vi "LIA Example FPGA_Original.vi"() -> ()   [LabVIEW 2017]
uses:
  <vilib>/eio/EIONode/EIONode.xnode
  <vilib>/rvi/eio/common/nirviEmuTemplateMethod_errors.vi
  <vilib>/Platform/TimedLoop/XDataNode/wakeup.ctl
  <vilib>/Platform/TimedLoop/XDataNode/XDNodeRunTimeDep.lvlib
  <vilib>/Platform/TimedLoop/XDataNode/nitl_modes.ctl
  <vilib>/Platform/TimedLoop/XDataNode/timing_clust.ctl
  <vilib>/Platform/TimedLoop/XDataNode/XDataNode.xnode
  <instrlib>/_niInstr/Basic Elements/v1/FPGA/niInstr Basic Elements v1 FPGA.lvlib
  <instrlib>/_niInstr/DSP/v1/Shared/Public/IQ Data.ctl
  <instrlib>/_niInstr/DSP/v1/Shared/niInstr DSP v1 Shared.lvlib
  <instrlib>/_niInstr/DSP/v1/FPGA/Public/Sub VIs/Frequency Shift/Frequency Shift - 1 spc.vi
  <instrlib>/_niInstr/DSP/v1/FPGA/niInstr DSP v1 FPGA.lvlib
  <instrlib>/_niInstr/DSP/v1/Xnodes/Public/Frequency Shift/niInstr DSP v1 Frequency Shift FPGA.xnode
  Program Files (x86)/National Instruments/LabVIEW 2017/examples/Lock-In Amplifier/_NI PLL IP/FPGA/NI PLL IP FPGA.lvlib
  <vilib>/rvi/FXPMathLib/FxpMul/XNode/nifxpmath_Multiplier.xnode
  <vilib>/rvi/FXPMathLib/FxpAdd/XNode/nifxpmath_Add.xnode
  <instrlib>/_niInstr/DSP/v1/FPGA/Public/Sub VIs/Frequency Shift/Frequency Shift - 2 spc.vi
  Program Files (x86)/National Instruments/LabVIEW 2017/examples/Lock-In Amplifier/lib/fpga/Lock-In Amplifier Example FPGA.lvlib
  <instrlib>/_niInstr/Streaming/v1/Common/Stream State.ctl
  <instrlib>/_niInstr/Streaming/v1/Common/niInstr Streaming v1 Common.lvlib
  <userlib>/_NI Noise Generation IP/FPGA/NI Noise Generation IP FPGA v2.lvlib
  <vilib>/rvi/FXPMathLib/sim/FxpSim.dll
  <userlib>/_NI Noise Generation IP/FPGA/Public/Low Level/AWGN FXP23x2.vi
panel:
  in  "lock-in.enable 3":bool
  in  "lock-in.enable 2":bool
  in  "lock-in.enable 1":bool
  in  "lock-in.carrier 3":fxp<+/-,48,0>
  in  "lock-in.carrier 2":fxp<+/-,48,0>
  in  "lock-in.enable 0":bool
  in  "lock-in.channel select 3":i32
  in  "lock-in.carrier select 3":i32
  in  "lock-in.cic config valid 3":bool
  in  "lock-in.cic config 3":cluster{"factor":fxp<+,16,16>, "shift":i16}
  in  "lock-in.reset 3":bool
  out "stream.state 3":T1 caption="stream.state 0"
  out "stream.samples transferred 3":u64 caption="stream.samples transferred 0"
  out "stream.metadata 3":u64 caption="stream.metadata 0"
  in  "stream.num samples 3":u64 caption="stream.num samples 0"
  in  "stream.request state 3":T1 caption="stream.request state 0"
  in  "lock-in.channel select 2":i32
  in  "lock-in.carrier select 2":i32
  in  "lock-in.cic config valid 2":bool
  in  "lock-in.cic config 2":cluster{"factor":fxp<+,16,16>, "shift":i16}
  in  "lock-in.reset 2":bool
  out "stream.state 2":T1 caption="stream.state 0"
  out "stream.samples transferred 2":u64 caption="stream.samples transferred 0"
  out "stream.metadata 2":u64 caption="stream.metadata 0"
  in  "stream.num samples 2":u64 caption="stream.num samples 0"
  in  "stream.request state 2":T1 caption="stream.request state 0"
  out "pll.vco output 0":fxp<+/-,48,0>
  out "pll.vco output 1":fxp<+/-,48,0>
  out "stream.metadata 4":u64 caption="stream.metadata 0"
  out "stream.samples transferred 4":u64 caption="stream.samples transferred 0"
  out "stream.state 4":T1 caption="stream.state 0"
  in  "stream.request state 4":T1 caption="stream.request state 0"
  in  "stream.num samples 4":u64 caption="stream.num samples 0"
  in  "preview.channel select":i32
  in  "ao.reset 3":bool
  in  "ao.carrier 2":fxp<+/-,48,0>=0.010000000000001563
  in  "ao.level 2":fxp<+/-,18,1>
  in  "ao.reset 2":bool
  in  "ao.carrier 1":fxp<+/-,48,0>=0.010000000000001563
  in  "ao.level 1":fxp<+/-,18,1>
  in  "ao.reset 1":bool
  in  "ao.reset 0":bool
  in  "ao.carrier 0":fxp<+/-,48,0>=0.010000000000001563
  in  "ao.level 0":fxp<+/-,18,1>
  in  "lock-in.channel select 1":i32
  in  "lock-in.channel select 0":i32
  in  "stream.request state 1":T1 caption="stream.request state 0"
  in  "stream.num samples 1":u64 caption="stream.num samples 0"
  out "stream.metadata 1":u64 caption="stream.metadata 0"
  out "stream.samples transferred 1":u64 caption="stream.samples transferred 0"
  out "stream.state 1":T1 caption="stream.state 0"
  in  "lock-in.reset 1":bool
  in  "lock-in.cic config 1":cluster{"factor":fxp<+,16,16>, "shift":i16}
  in  "lock-in.cic config valid 1":bool
  in  "lock-in.carrier select 1":i32
  in  "lock-in.carrier select 0":i32
  in  "lock-in.cic config valid 0":bool
  in  "lock-in.cic config 0":cluster{"factor":fxp<+,16,16>, "shift":i16}
  in  "lock-in.reset 0":bool
  in  "lock-in.carrier 1":fxp<+/-,48,0>
  in  "lock-in.carrier 0":fxp<+/-,48,0>
  in  "ao.level 3":fxp<+/-,18,1>
  in  "pll.channel 1":i32
  in  "pll.reset 1":bool
  in  "pll.enable 1":bool
  in  "pll.config 1":T2={"quiescent frequency"=0.10000000000000142, "compensation"=0.0, "psd gain"=-18, "loop filter"={"order"=4, "cutoff"=6}}
  in  "pll.channel 0":i32
  in  "ao.noise gain 3":fxp<+,18,1>=0.01000213623046875
  in  "ao.carrier 3":fxp<+/-,48,0>=0.010000000000001563
  in  "ao.noise seeds 3":fxp<+,23,23>[](array[numeric])=[1.0, 12323.0]
  in  "pll.reset 0":bool
  in  "pll.enable 0":bool
  in  "stream.request state 0":T1
  in  "stream.num samples 0":u64
  out "stream.metadata 0":u64
  out "stream.samples transferred 0":u64
  out "stream.state 0":T1
  in  "pll.config 0":T2={"quiescent frequency"=0.10000000000000142, "compensation"=0.0, "psd gain"=-18, "loop filter"={"order"=4, "cutoff"=6}}
  out "IO Module\\InitDone":bool
  out "IO Module\\User Error":u32
  in  "IO Module\\User Command":u32
  in  "IO Module\\User Command Valid":bool
  out "IO Module\\User Command Ready":bool
  in  "IO Module\\User Command Arg 0":u32
  in  "IO Module\\User Command Arg 1":u32
  out "IO Module\\User Command Error":u16
  out "IO Module\\User Command Return":u32
  out "IO Module\\User Command Return Valid":bool
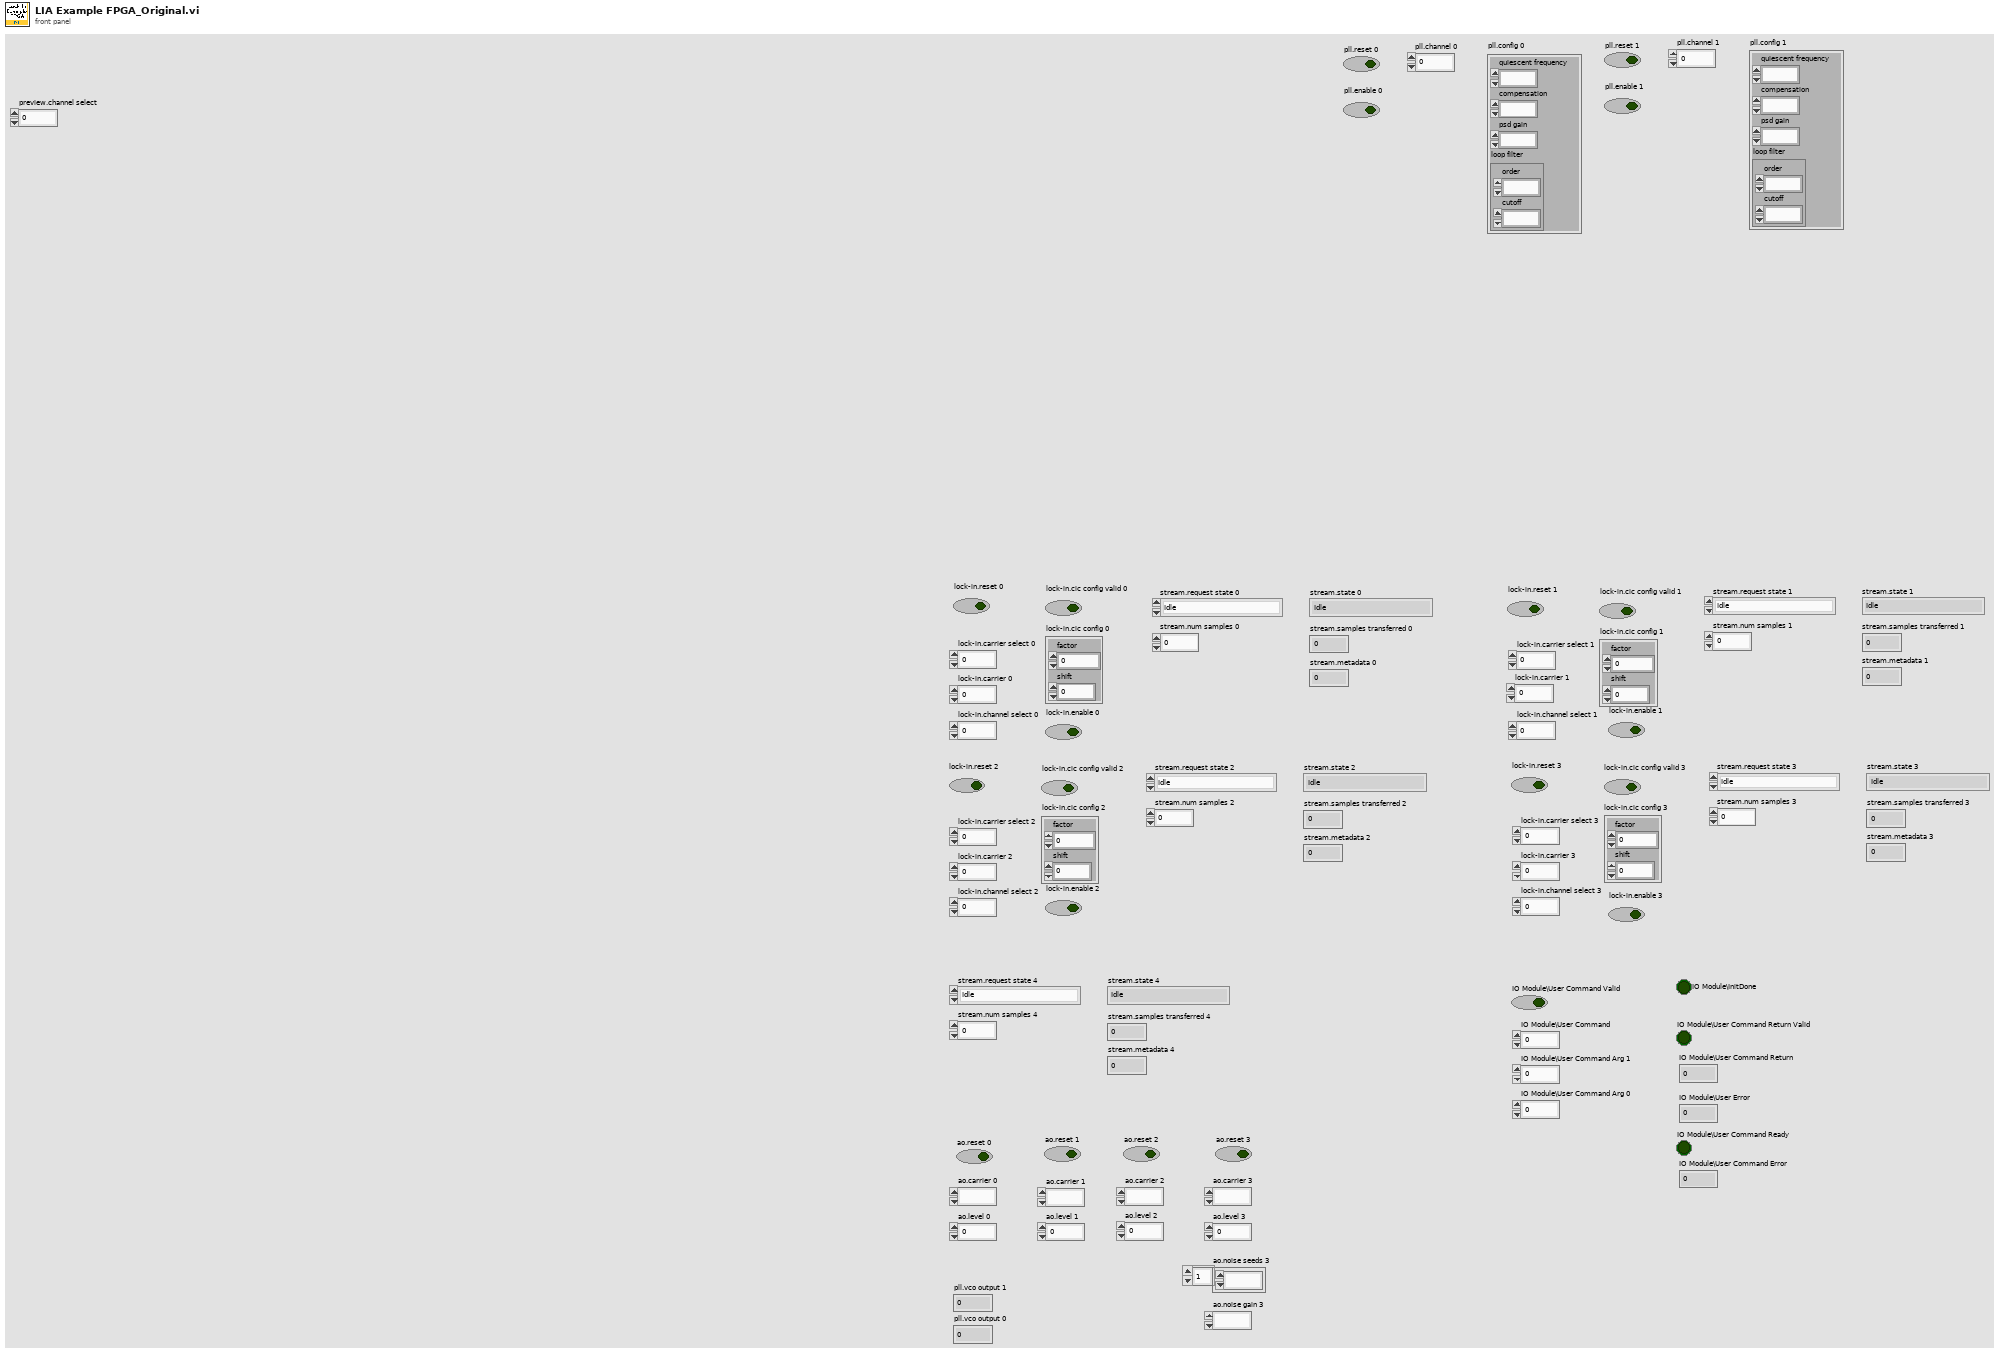
[diagram p1: front panel]
types:
  T1 = typedef "niInstr Streaming v1 Common.lvlib/Stream State.ctl" = enum8{"Idle", "Finite Transfer", "Continuous", "Done", "Error", "Not Ready", "Cancel"}
  T2 = cluster{"quiescent frequency":fxp<+/-,48,0>, "compensation":fxp<+/-,18,3>, "psd gain":i16, "loop filter":cluster{"order":i32, "cutoff":i8}}
  T3 = typedef "XDNodeRunTimeDep.lvlib/timing_clust.ctl" = cluster{"Expected End [f-1]":u64, "Actual End [f-1]":u64, "Finished Late? [f-1]":bool, "Expected End [i-1]":u64, "Actual End [i-1]":u64, "Finished Late? [i-1]":bool, "Expected Start [i]":u64, "Actual Start [i]":u64, "Expected Start [f]":u64, "Actual Start [f]":u64, "Source Name":string, "Structure Name":string, "Period":i64, "Deadline":i64, "Offset":i64, "Start":i64, "Priority":i32, "Timeout":i32, "Mode":T4, "Wakeup Reason":T5, "Error":errorcluster, "Source Type":string, "Secondary Source Type":string, "Global End Time":u64, "Global Start Time":u64, "Frame Duration":u64, "Iteration Duration":u64, "Assigned CPU":i32, "I/O Scan Engine Mode":u32}
  T4 = typedef "XDNodeRunTimeDep.lvlib/nitl_modes.ctl" = enum32{"No Change", "Process missed periods, maintain original phase", "Discard missed periods, maintain original phase", "Process missed periods, ignore original phase", "Discard missed periods, ignore original phase"}
  T5 = typedef "XDNodeRunTimeDep.lvlib/wakeup.ctl" = enum32{"Normal", "Aborted", "Asynchronous wakeup", "Timing source error", "Timed loop error", "Timeout"}
  T6 = cluster{"stream.num samples 0":u64, "stream.request state 0":T1, "stream.index 0":i16}
  T7 = typedef "niInstr DSP v1 Shared.lvlib/IQ Data.ctl" = cluster{"I":fxp<+/-,18,1>, "Q":fxp<+/-,18,1>, "overflow":bool}
  T8 = cluster{"stream.metadata 0":u64, "stream.samples transferred 0":u64, "stream.state 0":T1}
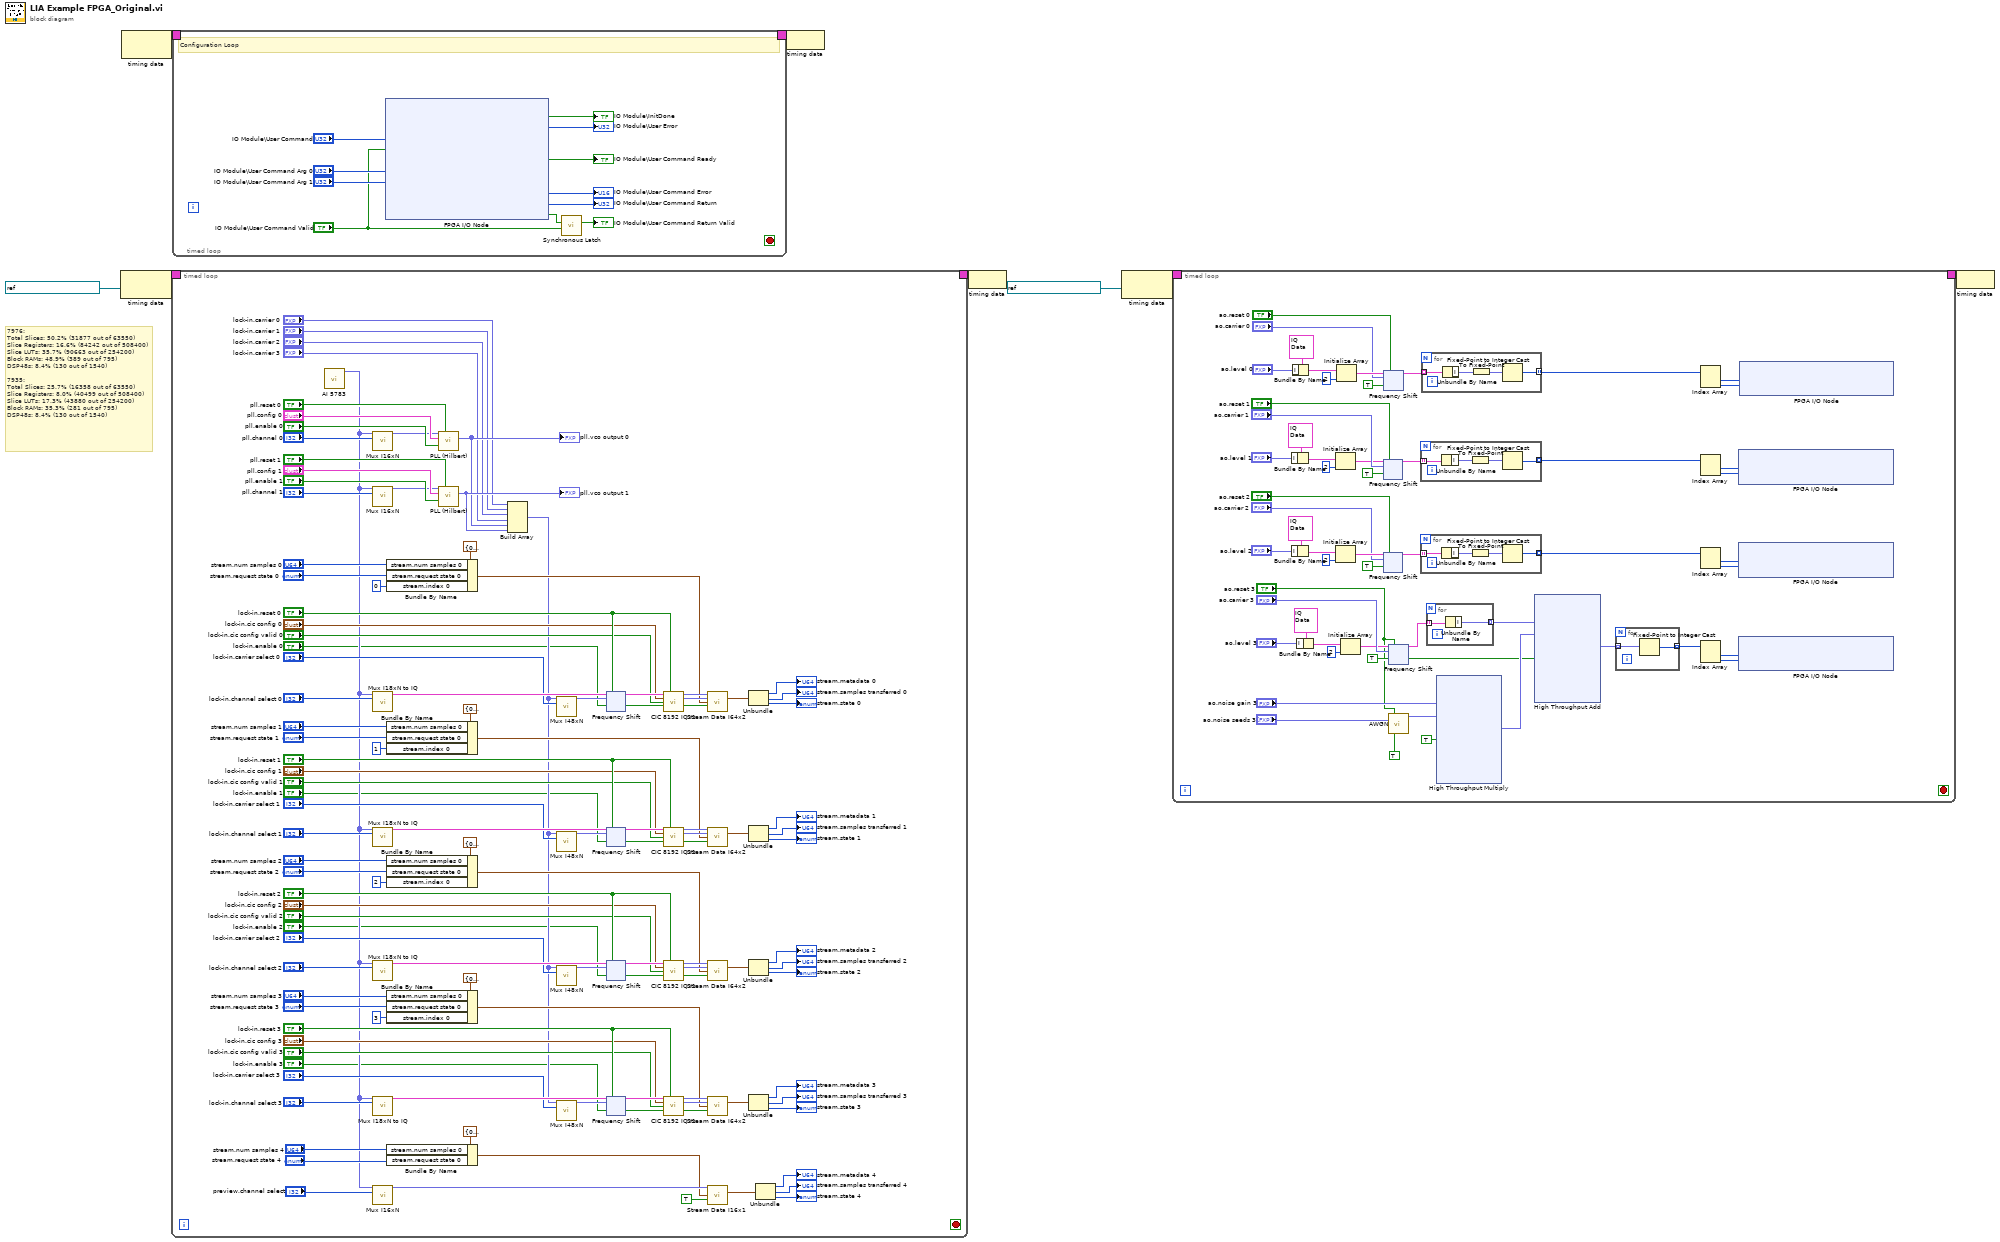
[diagram p0: block diagram]
diagram:
  # "7976:\nTotal Slices: 50.2% (31877 out of 63550)\nSlice Registers: 16.6% (84242 out of 508400)\nSlice LUTs: 35.7% (90663 out of 254200)\nBlock RAMs: 48.9% (389 out of 795)\nDSP48s: 8.4% (130 out of 1540)\n\n7935:\nTotal Slices: 25.7% (16358 out of 63550)\nSlice Registers: 8.0% (40499 out of 508400)\nSlice LUTs: 17.3% (43880 out of 254200)\nBlock RAMs: 35.3% (281 out of 795)\nDSP48s: 8.4% (130 out of 1540)"
  n1 = node-c288(refnum<k21> "IO Module\\Data Clock" ("Source Name")) -> (w8:T3)
  n2 = node-c288() -> (w2:T3)  [unwired: 1 in]
  n3 = timed-loop {
    timing: w8 -> [_]
    timing-out: [_] -> w7
    stop <- _ stop-if-true
    n4 = call "AI 5783.vi"() -> ("i18x1"=w17:fxp<+/-,18,1>[])  [unwired: 14 in, 1 out]
    n5 = call "Mux I16xN.vi"("i16xn in"=w17, "index"="pll.channel 0") -> ("i16 out"=w122:fxp<+/-,18,1>)  [unwired: 12 in, 1 out]
    n6 = call "Mux I16xN.vi"("i16xn in"=w17, "index"="pll.channel 1") -> ("i16 out"=w116:fxp<+/-,18,1>)  [unwired: 12 in, 1 out]
    n7 = call "Mux I18xN to IQ.vi"("i16xn in"=w17, "index"="lock-in.channel select 0") -> ("output"=w115:T7)  [unwired: 12 in, 1 out]
    n8 = call "Mux I18xN to IQ.vi"("i16xn in"=w17, "index"="lock-in.channel select 1") -> ("output"=w94:T7)  [unwired: 12 in, 1 out]
    n9 = call "Mux I18xN to IQ.vi"("i16xn in"=w17, "index"="lock-in.channel select 2") -> ("output"=w60:T7)  [unwired: 12 in, 1 out]
    n10 = call "Mux I18xN to IQ.vi"("i16xn in"=w17, "index"="lock-in.channel select 3") -> ("output"=w39:T7)  [unwired: 12 in, 1 out]
    n11 = call "Mux I16xN.vi"("i16xn in"=w17, "index"="preview.channel select") -> ("i16 out"=w68:fxp<+/-,18,1>)  [unwired: 12 in, 1 out]
    n12 = Bundle By Name(cluster=T6 {"stream.num samples 0"=0, "stream.request state 0"=enum."Idle", "stream.index 0"=0} ("config"), "stream.num samples 0"="stream.num samples 0", "stream.request state 0"="stream.request state 0", "stream.index 0"=i16 0) -> (w97:T6)
    n13 = Bundle By Name(cluster=T6 {"stream.num samples 0"=0, "stream.request state 0"=enum."Idle", "stream.index 0"=0} ("config"), "stream.num samples 0"="stream.num samples 1", "stream.request state 0"="stream.request state 1", "stream.index 0"=i16 1) -> (w76:T6)
    n14 = Bundle By Name(cluster=T6 {"stream.num samples 0"=0, "stream.request state 0"=enum."Idle", "stream.index 0"=0} ("config"), "stream.num samples 0"="stream.num samples 2", "stream.request state 0"="stream.request state 2", "stream.index 0"=i16 2) -> (w42:T6)
    n15 = Bundle By Name(cluster=T6 {"stream.num samples 0"=0, "stream.request state 0"=enum."Idle", "stream.index 0"=0} ("config"), "stream.num samples 0"="stream.num samples 3", "stream.request state 0"="stream.request state 3", "stream.index 0"=i16 3) -> (w21:T6)
    n16 = Bundle By Name(cluster=T6 {"stream.num samples 0"=0, "stream.request state 0"=enum."Idle", "stream.index 0"=0} ("config"), "stream.num samples 0"="stream.num samples 4", "stream.request state 0"="stream.request state 4") -> (w64:T6)
    n17 = call "PLL (Hilbert).vi"("input"=w122, "reset"="pll.reset 0", "config"="pll.config 0", "enable"="pll.enable 0") -> ("output"=w61:fxp<+/-,48,0>)  [unwired: 11 in]
    "pll.vco output 0" <- w61
    n18 = call "PLL (Hilbert).vi"("input"=w116, "reset"="pll.reset 1", "config"="pll.config 1", "enable"="pll.enable 1") -> ("output"=w62:fxp<+/-,48,0>)  [unwired: 11 in]
    "pll.vco output 1" <- w62
    n19 = Build Array("lock-in.carrier 0", "lock-in.carrier 1", "lock-in.carrier 2", "lock-in.carrier 3", w61, w62) -> (w18:fxp<+/-,48,0>[])
    n20 = call "Mux I48xN.vi"("i48xn in"=w18, "index"="lock-in.carrier select 0") -> ("i48 out"=w114:fxp<+/-,48,0>)  [unwired: 13 in]
    n21 = call "Mux I48xN.vi"("i48xn in"=w18, "index"="lock-in.carrier select 1") -> ("i48 out"=w93:fxp<+/-,48,0>)  [unwired: 13 in]
    n22 = call "Mux I48xN.vi"("i48xn in"=w18, "index"="lock-in.carrier select 2") -> ("i48 out"=w59:fxp<+/-,48,0>)  [unwired: 13 in]
    n23 = call "Mux I48xN.vi"("i48xn in"=w18, "index"="lock-in.carrier select 3") -> ("i48 out"=w38:fxp<+/-,48,0>)  [unwired: 13 in]
    n24 = xnode "Frequency Shift"("data in"=w115, "reset"="lock-in.reset 0", "frequency shift"=w114, "input valid"="lock-in.enable 0") -> ("data out"=w113:T7, "output valid"=w112:bool)  [unwired: 2 in, 1 out]
    n25 = xnode "Frequency Shift"("data in"=w94, "reset"="lock-in.reset 1", "frequency shift"=w93, "input valid"="lock-in.enable 1") -> ("data out"=w92:T7, "output valid"=w91:bool)  [unwired: 2 in, 1 out]
    n26 = xnode "Frequency Shift"("data in"=w60, "reset"="lock-in.reset 2", "frequency shift"=w59, "input valid"="lock-in.enable 2") -> ("data out"=w58:T7, "output valid"=w57:bool)  [unwired: 2 in, 1 out]
    n27 = xnode "Frequency Shift"("data in"=w39, "reset"="lock-in.reset 3", "frequency shift"=w38, "input valid"="lock-in.enable 3") -> ("data out"=w37:T7, "output valid"=w36:bool)  [unwired: 2 in, 1 out]
    n28 = call "CIC 8192 IQx1.vi"("data"=w113, "reset"="lock-in.reset 0", "config"="lock-in.cic config 0", "config valid"="lock-in.cic config valid 0", "input valid"=w112) -> ("i out"=w108:fxp<+/-,64,1>, "q out"=w107:fxp<+/-,64,1>, "output valid"=w106:bool)  [unwired: 8 in]
    n29 = call "CIC 8192 IQx1.vi"("data"=w92, "reset"="lock-in.reset 1", "config"="lock-in.cic config 1", "config valid"="lock-in.cic config valid 1", "input valid"=w91) -> ("i out"=w87:fxp<+/-,64,1>, "q out"=w86:fxp<+/-,64,1>, "output valid"=w85:bool)  [unwired: 8 in]
    n30 = call "CIC 8192 IQx1.vi"("data"=w58, "reset"="lock-in.reset 2", "config"="lock-in.cic config 2", "config valid"="lock-in.cic config valid 2", "input valid"=w57) -> ("i out"=w53:fxp<+/-,64,1>, "q out"=w52:fxp<+/-,64,1>, "output valid"=w51:bool)  [unwired: 8 in]
    n31 = call "CIC 8192 IQx1.vi"("data"=w37, "reset"="lock-in.reset 3", "config"="lock-in.cic config 3", "config valid"="lock-in.cic config valid 3", "input valid"=w36) -> ("i out"=w32:fxp<+/-,64,1>, "q out"=w31:fxp<+/-,64,1>, "output valid"=w30:bool)  [unwired: 8 in]
    n32 = call "Stream Data I64x2.vi"("i in"=w108, "q in"=w107, "config"=w97, "input valid"=w106) -> ("status"=w105:T8)  [unwired: 11 in]
    n33 = call "Stream Data I64x2.vi"("i in"=w87, "q in"=w86, "config"=w76, "input valid"=w85) -> ("status"=w84:T8)  [unwired: 11 in]
    n34 = call "Stream Data I64x2.vi"("i in"=w53, "q in"=w52, "config"=w42, "input valid"=w51) -> ("status"=w50:T8)  [unwired: 11 in]
    n35 = call "Stream Data I64x2.vi"("i in"=w32, "q in"=w31, "config"=w21, "input valid"=w30) -> ("status"=w29:T8)  [unwired: 11 in]
    n36 = call "Stream Data I16x1.vi"("i in"=w68, "config"=w64, "input valid"=TRUE) -> ("status"=w70:T8)  [unwired: 12 in]
    n37 = Unbundle(w105) -> ("stream.metadata 0"=→"stream.metadata 0":u64, "stream.samples transferred 0"=→"stream.samples transferred 0":u64, "stream.state 0"=→"stream.state 0":T1)
    n38 = Unbundle(w84) -> ("stream.metadata 0"=→"stream.metadata 1":u64, "stream.samples transferred 0"=→"stream.samples transferred 1":u64, "stream.state 0"=→"stream.state 1":T1)
    n39 = Unbundle(w50) -> ("stream.metadata 0"=→"stream.metadata 2":u64, "stream.samples transferred 0"=→"stream.samples transferred 2":u64, "stream.state 0"=→"stream.state 2":T1)
    n40 = Unbundle(w29) -> ("stream.metadata 0"=→"stream.metadata 3":u64, "stream.samples transferred 0"=→"stream.samples transferred 3":u64, "stream.state 0"=→"stream.state 3":T1)
    n41 = Unbundle(w70) -> ("stream.metadata 0"=→"stream.metadata 4":u64, "stream.samples transferred 0"=→"stream.samples transferred 4":u64, "stream.state 0"=→"stream.state 4":T1)
  }
  n42 = timed-loop {
    timing: w2 -> [_]
    timing-out: [_] -> w1
    stop <- _ stop-if-true
    # "Configuration Loop"
    n43 = xnode "FPGA I/O Node"("IO Module\\User Command"="IO Module\\User Command", "IO Module\\User Command Valid"="IO Module\\User Command Valid", "IO Module\\User Command Arg 0"="IO Module\\User Command Arg 0", "IO Module\\User Command Arg 1"="IO Module\\User Command Arg 1") -> ("IO Module\\InitDone"=→"IO Module\\InitDone":bool, "IO Module\\Clip Error Code"=→"IO Module\\User Error":u32, "IO Module\\User Command Ready"=→"IO Module\\User Command Ready":bool, "IO Module\\User Command Error"=→"IO Module\\User Command Error":u16, "IO Module\\User Command Return"=→"IO Module\\User Command Return":u32, "IO Module\\User Command Return Valid"=w165:bool)  [unwired: 10 in, 10 out]
    n44 = call <instrlib>:"Synchronous Latch.vi"("clear"="IO Module\\User Command Valid", "set"=w165) -> ("out"=→"IO Module\\User Command Return Valid":bool)  [unwired: 9 in]
  }
  n45 = node-c288(w1) -> ()
  n46 = node-c288(w7) -> ()
  n47 = node-c288(refnum<k21> "IO Module\\Data Clock" ("Source Name")) -> (w5:T3)
  n48 = timed-loop {
    timing: w5 -> [_]
    timing-out: [_] -> w4
    stop <- _ stop-if-true
    n49 = Bundle By Name(cluster=T7 {"I"=0.0, "Q"=0.0, "overflow"=FALSE} ("output"), "I"="ao.level 1") -> (w198:T7)
    n50 = Bundle By Name(cluster=T7 {"I"=0.0, "Q"=0.0, "overflow"=FALSE} ("output"), "I"="ao.level 2") -> (w188:T7)
    n51 = Bundle By Name(cluster=T7 {"I"=0.0, "Q"=0.0, "overflow"=FALSE} ("output"), "I"="ao.level 0") -> (w213:T7)
    n52 = Bundle By Name(cluster=T7 {"I"=0.0, "Q"=0.0, "overflow"=FALSE} ("output"), "I"="ao.level 3") -> (w222:T7)
    n53 = Initialize Array(w198, 2 ("dimension size")) -> (w194:T7[])
    n54 = Initialize Array(w188, 2 ("dimension size")) -> (w192:T7[])
    n55 = Initialize Array(w213, 2 ("dimension size")) -> (w217:T7[])
    n56 = Initialize Array(w222, 2 ("dimension size")) -> (w218:T7[])
    n57 = xnode "Frequency Shift"("data in"=w194, "reset"="ao.reset 1", "frequency shift"="ao.carrier 1", "input valid"=TRUE) -> ("data out"=w202:T7[])  [unwired: 2 in, 2 out]
    n58 = xnode "Frequency Shift"("data in"=w192, "reset"="ao.reset 2", "frequency shift"="ao.carrier 2", "input valid"=TRUE) -> ("data out"=w184:T7[])  [unwired: 2 in, 2 out]
    n59 = xnode "Frequency Shift"("data in"=w217, "reset"="ao.reset 0", "frequency shift"="ao.carrier 0", "input valid"=TRUE) -> ("data out"=w209:T7[])  [unwired: 2 in, 2 out]
    n60 = xnode "Frequency Shift"("data in"=w218, "reset"="ao.reset 3", "frequency shift"="ao.carrier 3", "input valid"=TRUE) -> ("data out"=w233:T7[], "output valid"=w230:bool)  [unwired: 2 in, 1 out]
    n61 = call-poly <userlib>:"AWGN.vi"("reset"="ao.reset 3", "seeds"="ao.noise seeds 3", "ready"=TRUE) -> ("output 0"=w225:fxp<+/-,23,4>[])  [unwired: 10 in, 2 out]
    n62 = for {
      tunnel: w202 -> [w249] mode=indexing
      tunnel: [w250] -> w203 mode=indexing
      n63 = Unbundle By Name(w249) -> ("I"=w248:fxp<+/-,18,1>)
      n64 = To Fixed-Point(number=w248) -> (fixed-point=w247:fxp<+/-,16,1>)  [unwired: 1 in]
      n65 = Fixed-Point to Integer Cast(1:w247) -> (0:w250:i16)
    }
    n66 = for {
      tunnel: w184 -> [w236] mode=indexing
      tunnel: [w237] -> w183 mode=indexing
      n67 = Unbundle By Name(w236) -> ("I"=w235:fxp<+/-,18,1>)
      n68 = To Fixed-Point(number=w235) -> (fixed-point=w234:fxp<+/-,16,1>)  [unwired: 1 in]
      n69 = Fixed-Point to Integer Cast(1:w234) -> (0:w237:i16)
    }
    n70 = for {
      tunnel: w209 -> [w262] mode=indexing
      tunnel: [w263] -> w208 mode=indexing
      n71 = Unbundle By Name(w262) -> ("I"=w261:fxp<+/-,18,1>)
      n72 = To Fixed-Point(number=w261) -> (fixed-point=w260:fxp<+/-,16,1>)  [unwired: 1 in]
      n73 = Fixed-Point to Integer Cast(1:w260) -> (0:w263:i16)
    }
    n74 = for {
      tunnel: w233 -> [w276] mode=indexing
      tunnel: [w275] -> w229 mode=indexing
      n75 = Unbundle By Name(w276) -> ("I"=w275:fxp<+/-,18,1>)
    }
    n76 = xnode ("High Throughput Multiply")("x"="ao.noise gain 3", "y"=w225, "input valid"=TRUE) -> ("x*y"=w232:fxp<+/-,41,5>[])  [unwired: 1 in, 2 out]
    n77 = xnode ("High Throughput Add")("x"=w229, "y"=w232, "input valid"=w230) -> ("x+y"=w224:fxp<+/-,16,1>[])  [unwired: 1 in, 2 out]
    n78 = for {
      tunnel: w224 -> [w274] mode=indexing
      tunnel: [w273] -> w193 mode=indexing
      n79 = Fixed-Point to Integer Cast(1:w274) -> (0:w273:i16)
    }
    n80 = Index Array(array=w208) -> (element #1=w207:i16, element #2=w206:i16)  [unwired: 2 in]
    n81 = Index Array(array=w203) -> (element #1=w204:i16, element #2=w205:i16)  [unwired: 2 in]
    n82 = Index Array(array=w183) -> (element #1=w182:i16, element #2=w181:i16)  [unwired: 2 in]
    n83 = Index Array(array=w193) -> (element #1=w180:i16, element #2=w179:i16)  [unwired: 2 in]
    n84 = xnode "FPGA I/O Node"("IO Module\\AO 1 Data N-1 Data Clock"=w204, "IO Module\\AO 1 Data N Data Clock"=w205) -> ()  [unwired: 2 in, 2 out]
    n85 = xnode "FPGA I/O Node"("IO Module\\AO 2 Data N-1 Data Clock"=w182, "IO Module\\AO 2 Data N Data Clock"=w181) -> ()  [unwired: 2 in, 2 out]
    n86 = xnode "FPGA I/O Node"("IO Module\\AO 3 Data N-1 Data Clock"=w180, "IO Module\\AO 3 Data N Data Clock"=w179) -> ()  [unwired: 2 in, 2 out]
    n87 = xnode "FPGA I/O Node"("IO Module\\AO 0 Data N-1 Data Clock"=w207, "IO Module\\AO 0 Data N Data Clock"=w206) -> ()  [unwired: 2 in, 2 out]
  }
  n88 = node-c288(w4) -> ()
